vi "Kick Global.vi"() -> ()   [LabVIEW 2013]
panel:
  in  "Cannon Info":T1
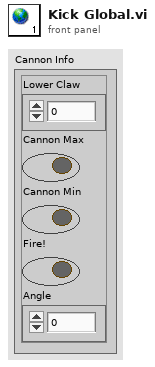
[diagram p1: front panel]
types:
  T1 = cluster{"Lower Claw":dbl, "Cannon Max":bool, "Cannon Min":bool, "Fire!":bool, "Angle":dbl}
diagram:
